vi "Stop Periodic Message.vi"(8 "error in":errorcluster, 11 "Chronometer in":refnum<class "Chronometer.lvclass">) -> (0 "error out":errorcluster, 3 "Chronometer out":refnum<class "Chronometer.lvclass">)   [LabVIEW 2023, in "Chronometer.lvlib" / "Chronometer.lvclass"]
uses:
  Chronometer.lvclass
  Chronometer.lvclass/Chronometer.ctl
  builds/Engine/Actor Framework.lvlibp/1abvi3w/vi.lib/ActorFramework/Time-Delayed Send Message/Time-Delay Override Options.ctl
  builds/Engine/Actor Framework.lvlibp
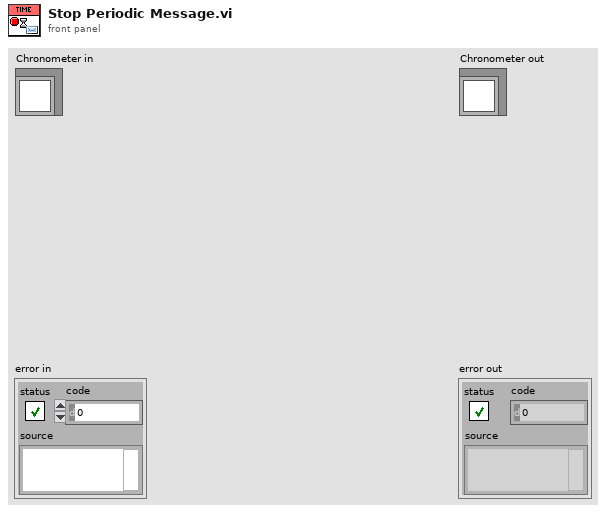
[diagram p1: front panel]
types:
  T1 = typedef "Actor Framework.lvlibp/Time-Delay Override Options.ctl" = enum16{"Send next copy now", "Skip next scheduled copy", "Send next copy now and stop all further copies", "Stop all further copies"}
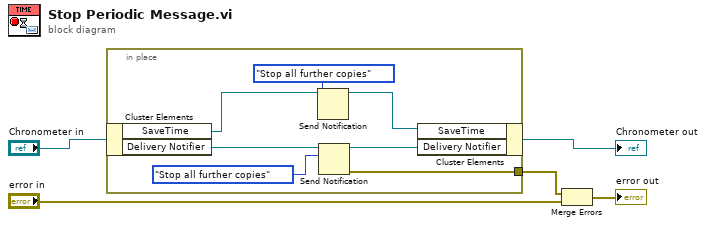
[diagram p0: block diagram]
diagram:
  n1 = in-place {
    in-place-border: [w9] -> w3
    n2 = in-place-cluster #1("Chronometer in") -> ("SaveTime"=w8:refnum<notifier>, "Delivery Notifier"=w11:refnum<notifier>)
    n3 = Send Notification(notification=Time-Delay_Override_Options."Stop all further copies", notifier=w8) -> (notifier out=w7:refnum<notifier>)  [unwired: 1 in, 1 out]
    n4 = Send Notification(notification=Time-Delay_Override_Options."Stop all further copies", notifier=w11) -> (notifier out=w10:refnum<notifier>, error out=w9:errorcluster)  [unwired: 1 in]
    n5 = in-place-cluster #1("SaveTime"=w7, "Delivery Notifier"=w10) -> (→"Chronometer out":refnum<class "Chronometer.lvclass">)
  }
  n6 = Merge Errors(w3, "error in") -> (→"error out":errorcluster)
